vi "make_url.vi"(3 "input cluster":T1) -> (7 "Url":string, 10 "input cluster 2":T1)   [LabVIEW 2019]
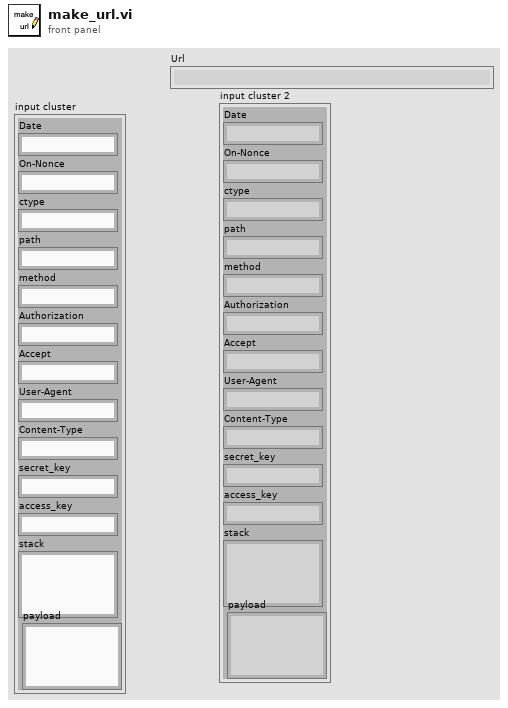
[diagram p1: front panel]
types:
  T1 = cluster{"Date":string, "On-Nonce":string, "ctype":string, "path":string, "method":string, "Authorization":string, "Accept":string, "User-Agent":string, "Content-Type":string, "secret_key":string, "access_key":string, "stack":string, "payload":string}
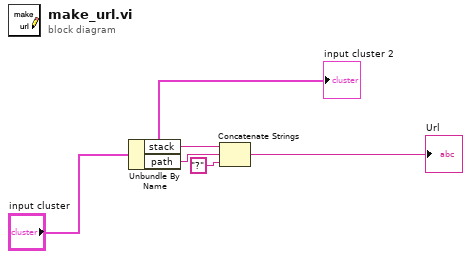
[diagram p0: block diagram]
diagram:
  n1 = Unbundle By Name("input cluster") -> ("stack"=w2:string, "path"=w3:string)
  n2 = Concatenate Strings(w2, w3, "?") -> (→"Url":string)
  "input cluster 2" <- "input cluster"
